vi "FFMPEG_Timestamp_Generator.vi"() -> ()   [LabVIEW 2020]
panel:
  out "error out":errorcluster
  out "UTC Timestamp Array":u64[](array[numeric])
  in  "Output txt File Path":path
  in  "Num of Frames to generate":u32=54000
  in  "Delta T (ns)":u64=1000000
  in  "Base Relative Time (ns)":u64=33333333
  in  "Timestamp Type":enum16{"Base", "Base +/- Rand(Delta T)"}(ring)
  in  "T0":timestamp=timestamp(3761082000 s since 1904-01-01)
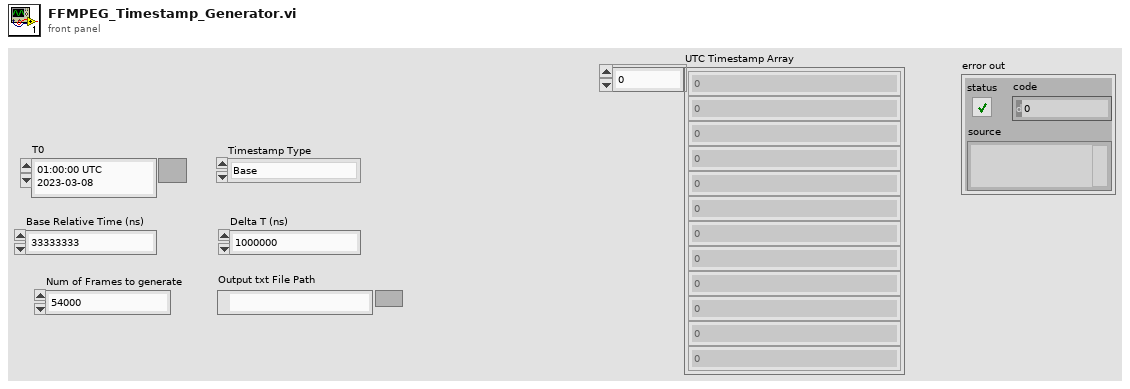
[diagram p1: front panel]
types:
  T1 = enum16{"open", "replace", "create", "open or create", "replace or create", "replace or create with confirmation"}
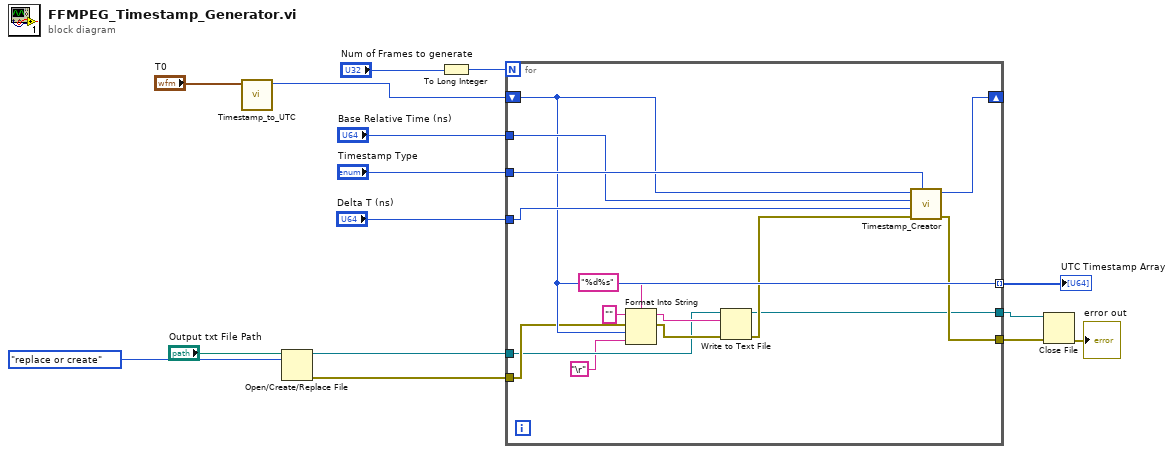
[diagram p0: block diagram]
diagram:
  n1 = call "Timestamp_to_UTC.vi"("Timestamp"="T0") -> ("UTC Time"=w9:u64)  [unwired: 9 in, 1 out]
  n2 = Open/Create/Replace File(file path (use dialog)="Output txt File Path", operation (0:open)=T1."replace or create") -> (refnum out=w4:refnum<file>, error out=w5:errorcluster)  [unwired: 4 in, 1 out]
  n3 = To Long Integer(number="Num of Frames to generate") -> (32bit integer=w14:i32)
  n4 = for {
    N: w14 -> [_]
    tunnel: "Base Relative Time (ns)" -> [w29]
    tunnel: "Timestamp Type" -> [w30]
    tunnel: "Delta T (ns)" -> [w28]
    shift-right: [w27] -> _
    shift-left: w9 -> [w26]
    tunnel: [w26] -> w8 mode=indexing
    tunnel: w5 -> [w25]
    tunnel: w4 -> [w22]
    tunnel: [w20] -> w3
    tunnel: [w19] -> w2
    n5 = Format Into String(format string="%d%s", initial string="", error in=w25, w26, "\r") -> (resulting string=w24:string, error out=w23:errorcluster)
    n6 = Write to Text File(file (use dialog)=w22, text=w24, error in=w23) -> (refnum out=w19:refnum<file>, error out=w21:errorcluster)  [unwired: 1 in, 1 out]
    n7 = call "Timestamp_Creator.vi"("Timestamp Type"=w30, "error in (no error)"=w21, "Delta T (ns)"=w28, "Base Relative Time (ns)"=w29, "Previous Time (ns)"=w26) -> ("error out"=w20:errorcluster, "Next Time (ns)"=w27:u64)  [unwired: 5 in]
  }
  "UTC Timestamp Array" <- w8
  n8 = Close File(refnum=w2, error in=w3) -> (error out=→"error out":errorcluster)  [unwired: 1 out]
